vi "EXDIR-YAML_Read_Dictionary.vi"() -> ()   [LabVIEW 2016]
panel:
  in  "hierarchy":string[](array[string])
  in  "tree-dictionary":cluster{"key":variant, "value":variant}[](array[cluster])
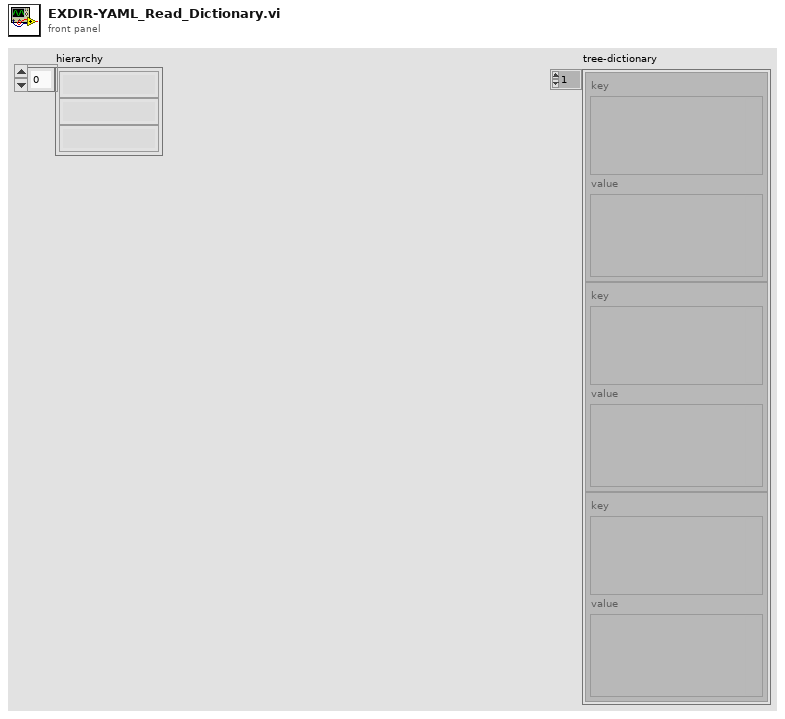
[diagram p1: front panel]
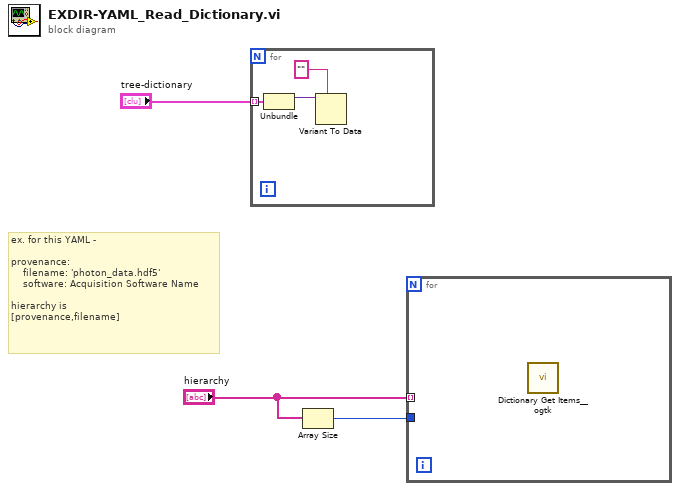
[diagram p0: block diagram]
diagram:
  # "ex. for this YAML -\n\nprovenance:\n    filename: 'photon_data.hdf5'\n    software: Acquisition Software Name\n\nhierarchy is \n[provenance,filename]"
  n1 = for {
    tunnel: "tree-dictionary" -> [w5] mode=indexing
    n2 = Unbundle(w5) -> ("key"=w4:variant)  [unwired: 1 out]
    n3 = Variant To Data(type="", Variant=w4) -> ()  [unwired: 1 in, 2 out]
  }
  n4 = Array Size(array="hierarchy") -> (size(s)=w2:i32)
  n5 = for {
    tunnel: "hierarchy" -> [_] mode=indexing
    tunnel: w2 -> [_]
    n6 = call <userlib>:"Dictionary Get Items__ogtk.vi"() -> ()  [unwired: 9 in, 3 out]
  }
